vi "Find Value in Key-Value Arrays.vi"(9 "Key Name":string, 10 "Values":refnum<class "Value.lvclass">[](array[class]), 11 "Keys":refnum<class "Key Name.lvclass">[](array[class])) -> (0 "Found?":bool, 1 "Value":refnum<class "Value.lvclass">, 2 "Values dup":refnum<class "Value.lvclass">[](array[class]), 3 "Keys dup":refnum<class "Key Name.lvclass">[](array[class]))   [LabVIEW 2019, in "Electronic Datasheet.lvlib"]
uses:
  Electronic Datasheet.lvlib
  Keyname/Key Name.lvclass
  Value/Value.lvclass
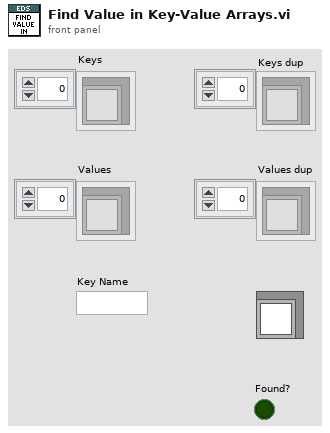
[diagram p1: front panel]
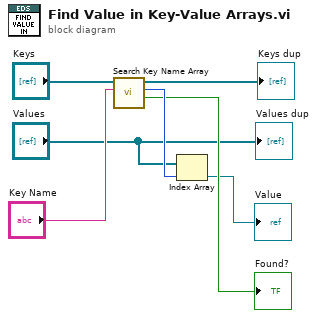
[diagram p0: block diagram]
diagram:
  n1 = call "Search Key Name Array.vi"("Key Name"="Key Name", "Keys"="Keys") -> ("Found?"=→"Found?":bool, "Index"=w5:i32, "Keys dup"=→"Keys dup":refnum<class "Key Name.lvclass">[])  [unwired: 7 in]
  n2 = Index Array(array="Values", index=w5) -> (element=→"Value":refnum<class "Value.lvclass">)
  "Values dup" <- "Values"
